vi "getAngle.vi"(6 "Channel":i32, 8 "error in (no error)":errorcluster, 11 "instrument.PPMS":refnum<class "instrument.PPMS.lvclass">) -> (0 "error out":errorcluster, 1 "Status":string, 2 "Angle (°)":dbl, 3 "instrument.PPMS out":refnum<class "instrument.PPMS.lvclass">, 4 "Finished?":bool)   [LabVIEW 2019, in "instrument.PPMS.lvclass"]
uses:
  instrument.PPMS.lvclass
  <userlib>/LevyLab/Instrument Framework/Instrument Types/Cryostat/Instrument.Cryostat.lvclass
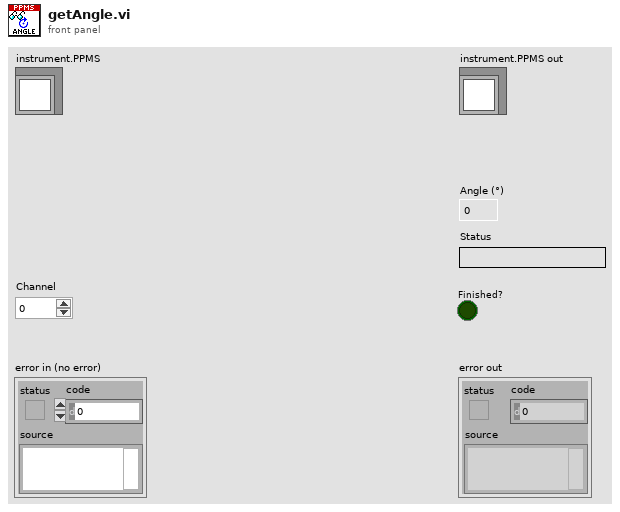
[diagram p1: front panel]
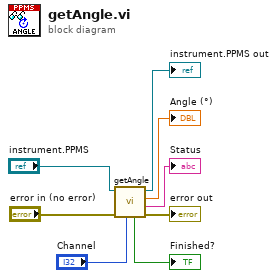
[diagram p0: block diagram]
diagram:
  n1 = call-parent "getAngle.vi"("Channel"="Channel", "error in (no error)"="error in (no error)", "Instrument.Cryostat in"="instrument.PPMS") -> ("error out"=→"error out":errorcluster, "Status"=→"Status":string, "Angle (°)"=→"Angle (°)":dbl, "Instrument.Cryostat out"=→"instrument.PPMS out":refnum<class "instrument.PPMS.lvclass">, "Finished?"=→"Finished?":bool)  [unwired: 4 in]
